vi "简单工厂+策略设计设计模式DEMO.vi"() -> ()   [LabVIEW 2013]
uses:
  Strategy_class/Operation Context.lvclass
  Operation_class/Operation.lvclass
  <vilib>/addons/_AddQ/G#Object/G#Object.lvclass
  Factory_class/Factory.lvclass
panel:
  in  "停止":bool
  out "# of objects killed":i32
  out "Output":string
  out "result":dbl
  in  "y":dbl
  in  "x":dbl
  in  "Operation":enum16{"Add", "Mul"}(ring)
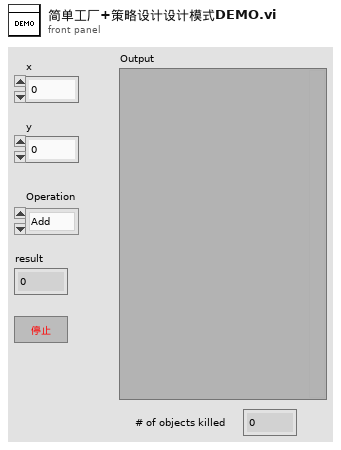
[diagram p1: front panel]
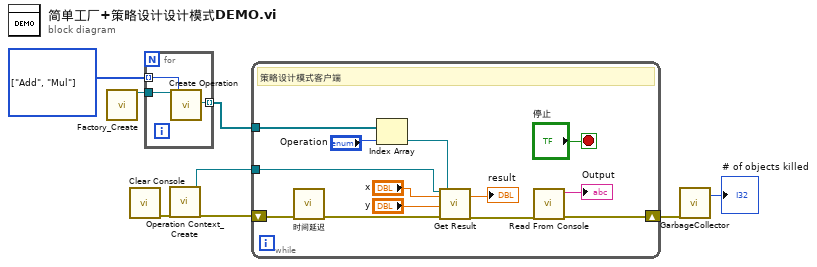
[diagram p0: block diagram]
diagram:
  w3 = enum16{"Add", "Mul"}[] [enum."Add", enum."Mul"] items=["Add", "Mul"]
  n1 = call "Factory_Create.vi"() -> ("reference out"=w2:refnum<class "Factory.lvclass">)  [unwired: 18 in, 1 out]
  n2 = call "Clear Console.vi"() -> ("error out"=w6:errorcluster)  [unwired: 11 in]
  n3 = for {
    tunnel: w3 -> [w10] mode=indexing
    tunnel: w2 -> [w11]
    tunnel: [w9] -> w1 mode=indexing
    n4 = call "Create Operation.vi"("reference in"=w11, "Operation"=w10) -> ("Operation"=w9:refnum<class "Operation.lvclass">)  [unwired: 15 in, 2 out]
  }
  n5 = call "Operation Context_Create.vi"("error in (no error)"=w6) -> ("reference out"=w4:refnum<class "Operation Context.lvclass">, "error out"=w5:errorcluster)  [unwired: 17 in]
  n6 = while {
    shift-right: [w23] -> w8
    shift-left: w5 -> [w24]
    tunnel: w4 -> [w16]
    tunnel: w1 -> [w19]
    stop <- "停止" stop-if-true
    # "策略设计模式客户端"
    n7 = call "时间延迟"("error in (no error)"=w24) -> ("error out"=w18:errorcluster)  [unwired: 10 in]
    n8 = Index Array(array=w19, index="Operation") -> (element=w15:refnum<class "Operation.lvclass">)
    n9 = call-dynamic "Get Result.vi"("reference in"=w16, "x"="x", "y"="y", "error in (no error)"=w18, "Operation.lvclass"=w15) -> ("result"=→"result":dbl, "error out"=w17:errorcluster)  [unwired: 12 in, 1 out]
    n10 = call "Read From Console.vi"("error in (no error)"=w17) -> ("error out"=w23:errorcluster, "Output"=→"Output":string)  [unwired: 9 in]
  }
  n11 = call <vilib>:"GarbageCollector.vi"("error in (no error)"=w8) -> ("# of objects killed"=→"# of objects killed":i32)  [unwired: 16 in, 2 out]
